vi "Start.vi"(8 "error in (no error)":errorcluster, 10 "Message in":refnum<class "StartMessage.lvclass">, 11 "DAQMH121119OrcaFlash in":refnum<class "DAQOrcaFlash.lvclass">) -> (0 "error out":errorcluster, 3 "DAQMH121119OrcaFlash out":refnum<class "DAQOrcaFlash.lvclass">)   [LabVIEW 2012, in "DAQOrcaFlash.lvclass"]
doc: "This member function is called when the statemachine in the run.vi receives an 'start' command. It relays the message to all observers of the component.\n\nOverride this member function in your derived class if you need additional start functionality (but don't forget to call the parent method)."
uses:
  DAQOrcaFlash.lvclass
  <vilib>/Distrio/Murmex/StartMessage/StartMessage.lvclass
  <vilib>/Distrio/Murmex/Murmex/Murmex.lvclass
  DAQOrcaFlash.lvclass/DAQOrcaFlash.ctl
  <vilib>/Distrio/Murmex/ProceedMessage/ProceedMessage.lvclass
  imaging_mode.ctl
  trigger_source.ctl
  trigger_mode.ctl
  <vilib>/Distrio/Murmex/GenericMessage/GenericMessage.lvclass
  <vilib>/Distrio/Murmex/Message/Add or replace parameter.vi
  <vilib>/Distrio/Murmex/ResetMessage/ResetMessage.lvclass
  <vilib>/Distrio/Murmex/Message/Message.lvclass
panel:
  # "This method is called when the START\ntrigger is sent. \n\nOverride this method when your component needs to\nrespond to this trigger. \n\nCall parent for proper implementation"
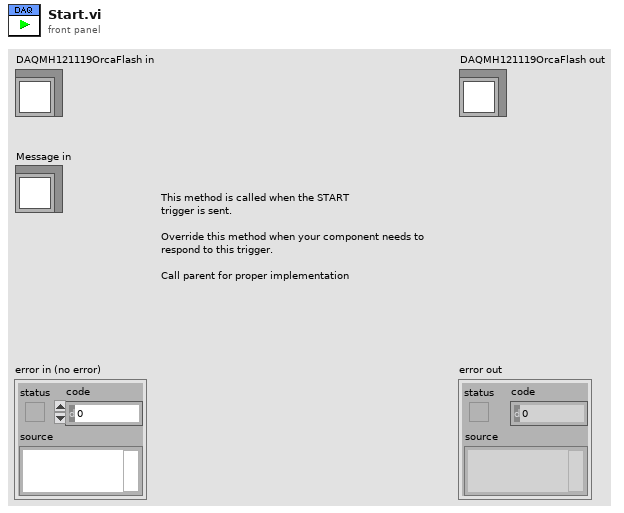
[diagram p1: front panel]
types:
  T1 = typedef "DAQOrcaFlash.lvclass/imaging_mode.ctl" = enum16{"focus mode", "single sweep"}
  T2 = typedef "Murmex.lvlib/StartMessage.lvclass/run mode enum.ctl" = enum16{"infinite", "finite"}
  T3 = typedef "DAQOrcaFlash.lvclass/trigger_mode.ctl" = sgl
  T4 = typedef "DAQOrcaFlash.lvclass/trigger_source.ctl" = sgl
  T5 = typedef "IMAQ Image.ctl" = refnum<image>
  T6 = cluster{"height":u32, "width":u32, "datatype":u32}
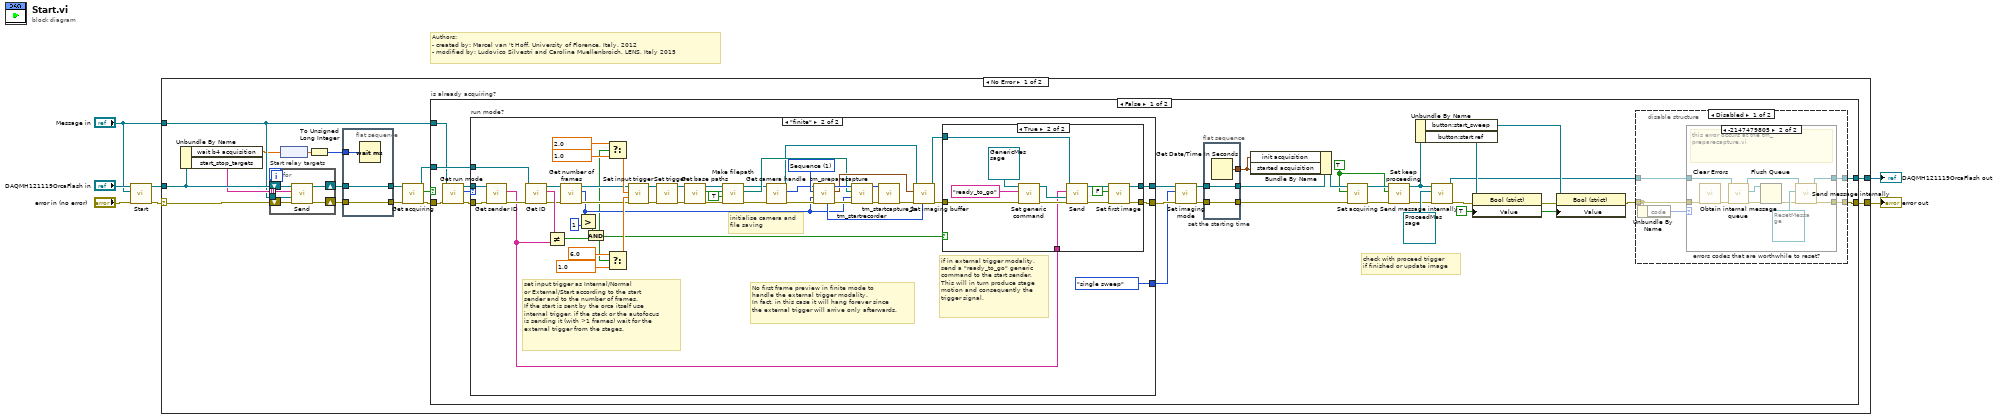
[diagram p0: block diagram]
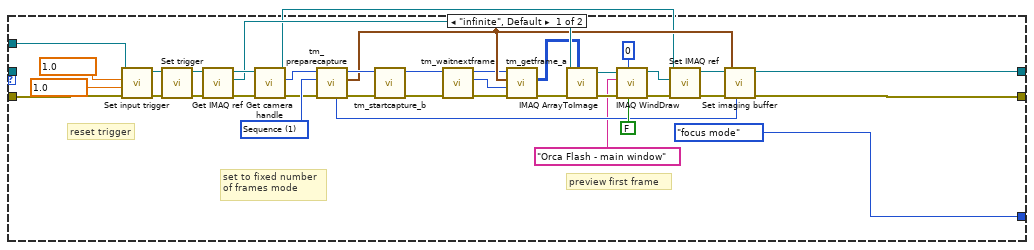
[diagram p4: hidden frame]
diagram:
  # "Authors: \n- created by: Marcel van 't Hoff, University of Florence, Italy, 2012\n- modified by: Ludovico Silvestri and Caroline Muellenbroich, LENS, Italy 2015"
  n1 = call-parent "Start.vi"("error in (no error)"="error in (no error)", "Message in"="Message in", "Murmex in"="DAQMH121119OrcaFlash in") -> ("error out"=w3:errorcluster, "Murmex out"=w4:refnum<class "DAQOrcaFlash.lvclass">)  [unwired: 7 in]
  n2 = case shown="No Error" w3 {
    selector: w3 -> [w16 w188]
    tunnel: [w23 w188] -> w2
    tunnel: [w22 w187] -> w7
    tunnel: w4 -> [w18 w187]
    tunnel: "Message in" -> [w11 _]
    frame No Error {
      n3 = Unbundle By Name(w18) -> ("wait b4 acquisition"=w10:dbl[unit], "start_stop_targets"=w17:string[])
      n4 = for "Start relay targets" {
        shift-right: [w32] -> w14
        shift-left: w16 -> [w31]
        tunnel: w11 -> [w29]
        tunnel: w17 -> [w28] mode=indexing
        shift-right: [w27] -> w12
        shift-left: w18 -> [w30]
        n5 = call <vilib>:"Send.vi"("error in (no error)"=w31, "Message"=w29, "recipient"=w28, "Murmex in"=w30) -> ("error out"=w32:errorcluster, "Murmex out"=w27:refnum<class "DAQOrcaFlash.lvclass">)  [unwired: 6 in]
      }
      n6 = node(w10) -> (w9:dbl)
      n7 = To Unsigned Long Integer(number=w9) -> (unsigned 32bit integer=w8:u32)
      n8 = flat-sequence {
        tunnel: [w26] -> w15
        tunnel: w14 -> [w26]
        tunnel: [w25] -> w13
        tunnel: w12 -> [w25]
        tunnel: w8 -> [w24]
        frame #0 {
          n9 = Wait (ms)(milliseconds to wait=w24) -> ()  [unwired: 1 out]
        }
      }
      n10 = call "Get acquiring.vi"("error in (no error)"=w15, "DAQMH121119OrcaFlash in"=w13) -> ("error out"=w20:errorcluster, "is acquiring?"=w19:bool, "DAQMH121119OrcaFlash out"=w21:refnum<class "DAQOrcaFlash.lvclass">)  [unwired: 7 in]
      n11 = case "is already acquiring?" shown="False" w19 {
        tunnel: [w42 w186] -> w23
        tunnel: [w39 w185] -> w22
        tunnel: w21 -> [w53 w185]
        tunnel: w20 -> [w46 w186]
        tunnel: w11 -> [w43 _]
        frame False {
          w56 = TRUE ("Value")
          w33 = TRUE ("is acquiring?")
          # "check with proceed trigger\nif finished or update image"
          n12 = call <vilib>:"Get run mode.vi"("error in (no error)"=w46, "StartMessage in"=w43) -> ("error out"=w45:errorcluster, "run mode"=w44:T2, "StartMessage out"=w37:refnum<class "StartMessage.lvclass">)  [unwired: 7 in]
          n13 = case "run mode?" shown="\"finite\"" w44 {
            tunnel: w45 -> [w89 w154]
            tunnel: [w119 w127] -> w62
            tunnel: [w120 w125] -> w51
            tunnel: w53 -> [w90 w155]
            tunnel: [imaging_mode."focus mode" ("imaging mode") imaging_mode."single sweep" ("imaging mode")] -> w49
            tunnel: w37 -> [_ w152]
            frame "infinite", Default {
              w85 = T3 1.0 items=["Normal"=1.0, "Start"=6.0] ("Trigger mode")
              w86 = T4 1.0 items=["Internal"=1.0, "External"=2.0, "Software"=3.0] ("Trigger source")
              w112 = 1 items=["Snap", "Sequence"] ("Capture mode")
              # "reset trigger"
              # "preview first frame"
              # "set to fixed number\nof frames mode"
              n14 = call-dynamic "Set input trigger.vi"("error in (no error)"=w89, "Trigger mode"=w85, "Trigger source"=w86, "DAQOrcaFlash in"=w90) -> ("error out"=w88:errorcluster, "DAQOrcaFlash out"=w91:refnum<class "DAQOrcaFlash.lvclass">)  [unwired: 6 in]
              n15 = call-dynamic "Set trigger.vi"("error in (no error)"=w88, "DAQOrcaFlash in"=w91) -> ("error out"=w87:errorcluster, "DAQOrcaFlash out"=w92:refnum<class "DAQOrcaFlash.lvclass">)  [unwired: 8 in]
              n16 = call "Get IMAQ ref.vi"("error in (no error)"=w87, "DAQMH121119OrcaFlash in"=w92) -> ("error out"=w121:errorcluster, "IMAQ reference"=w106:T5, "DAQMH121119OrcaFlash out"=w122:refnum<class "DAQOrcaFlash.lvclass">)  [unwired: 7 in]
              n17 = call "Get camera handle.vi"("error in (no error)"=w121, "DAQMH121119OrcaFlash in"=w122) -> ("error out"=w95:errorcluster, "cam handle"=w96:u32, "DAQMH121119OrcaFlash out"=w99:refnum<class "DAQOrcaFlash.lvclass">)  [unwired: 7 in]
              n18 = call <userlib>:"tm_preparecapture.vi"("error in (no error)"=w95, "Capture mode"=w112, "Handle in"=w96) -> ("error out"=w113:errorcluster, "Buffer Info"=w104:T6, "Handle out"=w111:u32, "Image type"=w103:u32)  [unwired: 5 in]
              n19 = call <userlib>:"tm_startcapture_b.vi"("error in (no error)"=w113, "Handle in"=w111) -> ("error out"=w109:errorcluster, "Handle out"=w110:u32)  [unwired: 8 in]
              n20 = call <userlib>:"tm_waitnextframe.vi"("error in (no error)"=w109, "Handle in"=w110) -> ("error out"=w94:errorcluster, "Frame Index"=w108:i32, "Handle out"=w93:u32)  [unwired: 6 in, 1 out]
              n21 = call <userlib>:"tm_getframe_a.vi"("error in (no error)"=w94, "Frame Index"=w108, "Buffer Info"=w104, "Handle in"=w93) -> ("error out"=w100:errorcluster, "Data 16"=w102:u16[][])  [unwired: 3 in, 3 out]
              n22 = call "IMAQ ArrayToImage"("Image Pixels (U16)"=w102, "error in (no error)"=w100, "Image"=w106) -> ("error out"=w107:errorcluster, "Image Out"=w105:T5)  [unwired: 7 in]
              n23 = call "IMAQ WindDraw"("Resize to Image Size? (Y)"=FALSE, "Window Number (0...15)"=0, "error in (no error)"=w107, "Title"="Orca Flash - main window", "Image"=w105) -> ("error out"=w115:errorcluster, "Image Out (duplicate)"=w101:T5)  [unwired: 5 in]
              n24 = call "Set IMAQ ref.vi"("error in (no error)"=w115, "IMAQ reference"=w101, "DAQMH121119OrcaFlash in"=w99) -> ("error out"=w116:errorcluster, "DAQMH121119OrcaFlash out"=w117:refnum<class "DAQOrcaFlash.lvclass">)  [unwired: 7 in]
              n25 = call "Set imaging buffer.vi"("Image type"=w103, "error in (no error)"=w116, "Buffer"=w104, "DAQMH121119OrcaFlash in"=w117) -> ("error out"=w119:errorcluster, "DAQMH121119OrcaFlash out"=w120:refnum<class "DAQOrcaFlash.lvclass">)  [unwired: 6 in]
            }
            frame "finite" {
              w142 = T3 1.0 items=["Normal"=1.0, "Start"=6.0] ("Trigger mode")
              w143 = T3 6.0 items=["Normal"=1.0, "Start"=6.0] ("Trigger mode")
              w146 = T4 1.0 items=["Internal"=1.0, "External"=2.0, "Software"=3.0] ("Trigger source")
              w145 = T4 2.0 items=["Internal"=1.0, "External"=2.0, "Software"=3.0] ("Trigger source")
              w168 = 1 items=["Snap", "Sequence"] ("Capture mode")
              # "if in external trigger modality,\nsend a \"ready_to_go\" generic\ncommand to the start sender.\nThis will in turn produce stage\nmotion and consequently the\ntrigger signal."
              # "No first frame preview in finite mode to\nhandle the external trigger modality.\nIn fact, in this case it will hang forever since\nthe external trigger will arrive only afterwards."
              # "set input trigger as Internal/Normal\nor External/Start according to the start\nsender and to the number of frames.\nIf the start is sent by the orca itself use\ninternal trigger, if the stack or the autofocus\nis sending it (with >1 frames) wait for the \nexternal trigger from the stages."
              # "initialise camera and\nfile saving"
              n26 = call <vilib>:"Get sender ID.vi"("error in (no error)"=w154, "Message in"=w152) -> ("error out"=w153:errorcluster, "sender"=w124:string)  [unwired: 7 in, 1 out]
              n27 = call <vilib>:"Get ID.vi"("error in (no error)"=w153, "Murmex in"=w155) -> ("error out"=w138:errorcluster, "component id"=w151:string, "Murmex out"=w140:refnum<class "DAQOrcaFlash.lvclass">)  [unwired: 7 in]
              n28 = Not Equal?(x=w151, y=w124) -> (x != y?=w132:bool)
              n29 = call "Get number of frames.vi"("error in (no error)"=w138, "DAQMH121119OrcaFlash in"=w140) -> ("error out"=w137:errorcluster, "no. of frames"=w134:i32, "DAQMH121119OrcaFlash out"=w139:refnum<class "DAQOrcaFlash.lvclass">)  [unwired: 7 in]
              n30 = Greater?(x=w134, y=1) -> (0:w131:bool)
              n31 = And(x=w131, y=w132) -> (x .and. y?=w123:bool)
              n32 = Select(t=w145, s=w123, f=w146) -> (s? t:f=w144:T4)
              n33 = Select(t=w143, s=w123, f=w142) -> (s? t:f=w141:T3)
              n34 = call-dynamic "Set input trigger.vi"("error in (no error)"=w137, "Trigger mode"=w141, "Trigger source"=w144, "DAQOrcaFlash in"=w139) -> ("error out"=w147:errorcluster, "DAQOrcaFlash out"=w148:refnum<class "DAQOrcaFlash.lvclass">)  [unwired: 6 in]
              n35 = call-dynamic "Set trigger.vi"("error in (no error)"=w147, "DAQOrcaFlash in"=w148) -> ("error out"=w150:errorcluster, "DAQOrcaFlash out"=w149:refnum<class "DAQOrcaFlash.lvclass">)  [unwired: 8 in]
              n36 = call-dynamic "Get base paths.vi"("error in (no error)"=w150, "DAQOrcaFlash in"=w149) -> ("error out"=w164:errorcluster, "filepath"=w162:path, "DAQOrcaFlash out"=w163:refnum<class "DAQOrcaFlash.lvclass">)  [unwired: 6 in, 1 out]
              n37 = call "Make filepath.vi"("error in (no error)"=w164, "is cxd file path?"=TRUE, "base path"=w162, "DAQOrcaFlash in"=w163) -> ("error out"=w135:errorcluster, "filepath out"=w161:path, "DAQOrcaFlash out"=w136:refnum<class "DAQOrcaFlash.lvclass">)  [unwired: 5 in]
              n38 = call "Get camera handle.vi"("error in (no error)"=w135, "DAQMH121119OrcaFlash in"=w136) -> ("error out"=w157:errorcluster, "cam handle"=w158:u32, "DAQMH121119OrcaFlash out"=w129:refnum<class "DAQOrcaFlash.lvclass">)  [unwired: 7 in]
              n39 = call <userlib>:"tm_preparecapture.vi"("error in (no error)"=w157, "Frames"=w134, "Capture mode"=w168, "Handle in"=w158) -> ("error out"=w169:errorcluster, "Buffer Info"=w165:T6, "Handle out"=w170:u32, "Image type"=w166:u32)  [unwired: 4 in]
              n40 = call <userlib>:"tm_startrecorder.vi"("error in (no error)"=w169, "frames"=w134, "File"=w161, "Handle in"=w170) -> ("error out"=w159:errorcluster, "Handle out"=w160:u32)  [unwired: 6 in]
              n41 = call <userlib>:"tm_startcapture_b.vi"("error in (no error)"=w159, "Handle in"=w160) -> ("error out"=w130:errorcluster)  [unwired: 8 in, 1 out]
              n42 = call "Set imaging buffer.vi"("Image type"=w166, "error in (no error)"=w130, "Buffer"=w165, "DAQMH121119OrcaFlash in"=w129) -> ("error out"=w128:errorcluster, "DAQMH121119OrcaFlash out"=w126:refnum<class "DAQOrcaFlash.lvclass">)  [unwired: 6 in]
              n43 = case shown="True" w123 {
                tunnel: w128 -> [w171 w183]
                tunnel: [w171 w176] -> w127
                tunnel: w126 -> [w172 w181]
                tunnel: [w172 w174] -> w125
                tunnel: w124 -> [_ w178]
                frame False {
                }
                frame True {
                  n44 = call <vilib>:"Set generic command.vi"("error in (no error)"=w183, "generic command"="ready_to_go", "GenericMessage in"=refnum<class "GenericMessage.lvclass"> refnum ("Distrio Murmex 1.2:GenericMessage")) -> ("error out"=w184:errorcluster, "GenericMessage out"=w179:refnum<class "GenericMessage.lvclass">)  [unwired: 7 in]
                  n45 = call <vilib>:"Send.vi"("error in (no error)"=w184, "Message"=w179, "recipient"=w178, "Murmex in"=w181) -> ("error out"=w182:errorcluster, "Murmex out"=w175:refnum<class "DAQOrcaFlash.lvclass">)  [unwired: 6 in]
                  n46 = call-dynamic "Set first image.vi"("error in (no error)"=w182, "first image acquired?"=FALSE, "DAQOrcaFlash in"=w175) -> ("error out"=w176:errorcluster, "DAQOrcaFlash out"=w174:refnum<class "DAQOrcaFlash.lvclass">)  [unwired: 7 in]
                }
              }
            }
          }
          n47 = call "Set imaging mode.vi"("error in (no error)"=w62, "imaging mode"=w49, "DAQMH121119OrcaFlash in"=w51) -> ("error out"=w52:errorcluster, "DAQMH121119OrcaFlash out"=w50:refnum<class "DAQOrcaFlash.lvclass">)  [unwired: 7 in]
          n48 = flat-sequence "set the starting time" {
            tunnel: [w84] -> w59
            tunnel: w50 -> [w84]
            tunnel: w52 -> [w83]
            tunnel: [w83] -> w61
            tunnel: [w82] -> w38
            frame #0 {
              n49 = Get Date/Time In Seconds() -> (seconds since 1Jan1904=w82:timestamp)
            }
          }
          n50 = Bundle By Name(cluster=w59, "init acquisition"=w38, "started acquisition"=w38) -> (w60:refnum<class "DAQOrcaFlash.lvclass">)
          n51 = call "Set acquiring.vi"("error in (no error)"=w61, "is acquiring?"=w33, "DAQMH121119OrcaFlash in"=w60) -> ("error out"=w48:errorcluster, "DAQMH121119OrcaFlash out"=w35:refnum<class "DAQOrcaFlash.lvclass">)  [unwired: 7 in]
          n52 = call-dynamic "Set keep proceeding.vi"("error in (no error)"=w48, "keep proceeding?"=w33, "DAQOrcaFlash in"=w35) -> ("error out"=w36:errorcluster, "DAQOrcaFlash out"=w34:refnum<class "DAQOrcaFlash.lvclass">)  [unwired: 7 in]
          n53 = Unbundle By Name(w34) -> ("button:start_sweep"=w54:refnum<vi>, "button:start ref"=w58:refnum<vi>)
          n54 = call <vilib>:"Send message internally.vi"("error in (no error)"=w36, "Message"=refnum<class "ProceedMessage.lvclass"> refnum ("ProceedMessage"), "Murmex in"=w34) -> ("error out"=w57:errorcluster, "Murmex out"=w40:refnum<class "DAQOrcaFlash.lvclass">)  [unwired: 7 in]
          n55 = property class="Bool (strict)"(reference=w58, error in=w57, "Value"=w56) -> (error out=w55:errorcluster)  [unwired: 1 out]
          n56 = property class="Bool (strict)"(reference=w54, error in=w55, "Value"=w56) -> (error out=w41:errorcluster)  [unwired: 1 out]
          n57 = disable-structure shown="Disabled" {
            disable-tunnel: [w67 w80] -> w42
            disable-tunnel: w41 -> [w66 w80]
            disable-tunnel: w40 -> [w65 w81]
            disable-tunnel: [w64 w81] -> w39
            frame Disabled {
              n58 = Unbundle By Name(w66) -> ("code"=w63:i32)
              n59 = case "errors codes that are worthwhile to reset?" shown="-2147479805" w63 {
                tunnel: [w69 w78] -> w67
                tunnel: w66 -> [w69 w79]
                tunnel: w65 -> [w68 w75]
                tunnel: [w68 w77] -> w64
                frame Default {
                }
                frame -2147479805 {
                  # "this error occurs at the tm_preparecapture.vi"
                  n60 = call <vilib>:"Clear Errors.vi"("error in (no error)"=w79) -> ("error out"=w74:errorcluster)  [unwired: 6 in]
                  n61 = call <vilib>:"Obtain internal message queue.vi"("error in (no error)"=w74, "Murmex in"=w75) -> ("error out"=w71:errorcluster, "internal message queue"=w72:refnum<queue>, "Murmex out"=w73:refnum<class "DAQOrcaFlash.lvclass">)  [unwired: 7 in]
                  n62 = Flush Queue(queue=w72, error in (no error)=w71) -> (error out=w70:errorcluster)  [unwired: 2 out]
                  n63 = call <vilib>:"Send message internally.vi"("error in (no error)"=w70, "Message"=refnum<class "ResetMessage.lvclass"> refnum ("Message in"), "Murmex in"=w73) -> ("error out"=w78:errorcluster, "Murmex out"=w77:refnum<class "DAQOrcaFlash.lvclass">)  [unwired: 7 in]
                }
              }
            }
            frame Enabled {
            }
          }
        }
        frame True {
          # "Skip double start trigger events"
        }
      }
    }
    frame Error {
    }
  }
  "DAQMH121119OrcaFlash out" <- w7
  "error out" <- w2
